vi "Main.vi"(0 "Operations":string(tree), 5 "Path":path=path "C:/Users/khishore.kumar/Khishore/Assignment backups/Assignment 23/SubVI", 7 "Show":bool, 9 "Stop":bool, 11 "Error in":errorcluster) -> (15 "Error out":errorcluster)   [LabVIEW 2020, in "Subpanel access.lvlib"]
doc: "This system will have a file hierarchy to and on double click the panel will be displayed on the subpanel"
uses:
  Subpanel access.lvlib
panel:
  # "SUBPANEL ACCESS"
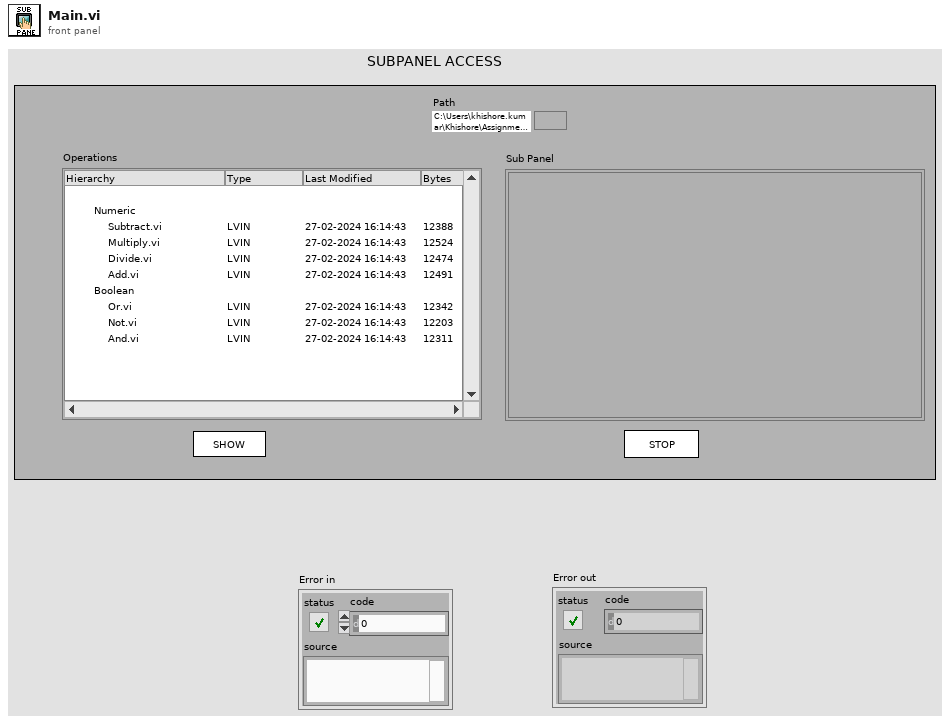
[diagram p1: front panel]
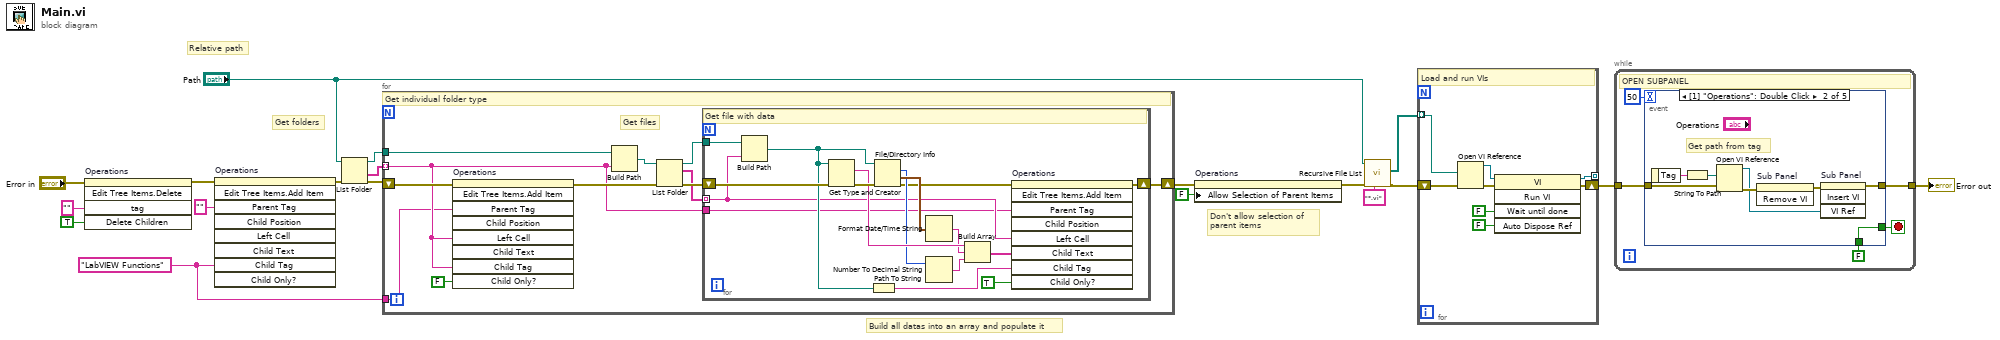
[diagram p0: block diagram]
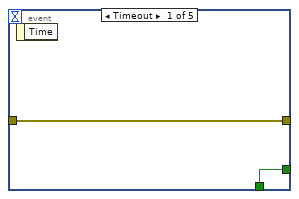
[diagram p2: hidden frame]
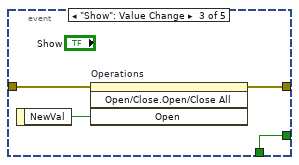
[diagram p3: hidden frame]
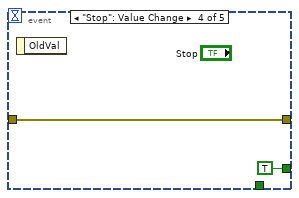
[diagram p4: hidden frame]
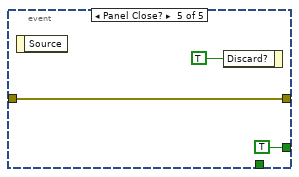
[diagram p5: hidden frame]
diagram:
  w2 = "LabVIEW Functions" ("Child Tag")
  # "Get folders"
  # "Build all datas into an array and populate it"
  # "Relative path"
  # "Don't allow selection of \nparent items"
  n1 = invoke on="Operations" class="Tree (strict)" method="Edit Tree Items.Delete"(error in="Error in", "tag"="" ("Tag"), "Delete Children"=TRUE ("Delete Children?")) -> (error out=w6:errorcluster)  [unwired: 2 in, 4 out]
  n2 = invoke on="Operations" class="Tree (strict)" method="Edit Tree Items.Add Item"(error in=w6, "Parent Tag"="", "Child Tag"=w2) -> (error out=w7:errorcluster)  [unwired: 6 in, 8 out]
  n3 = List Folder(path="Path", error in=w7) -> (path out=w14:path, folder names=w13:string[], error out=w12:errorcluster)  [unwired: 2 in, 1 out]
  n4 = for {
    tunnel: w14 -> [w29]
    shift-right: [w30] -> w5
    shift-left: w12 -> [w23]
    tunnel: w13 -> [w22] mode=indexing
    tunnel: w2 -> [w21]
    # "Get files"
    # "Get individual folder type"
    n5 = invoke on="Operations" class="Tree (strict)" method="Edit Tree Items.Add Item"(error in=w23, "Parent Tag"=w21, "Left Cell"=w22, "Child Tag"=w22, "Child Only?"=FALSE) -> (error out=w24:errorcluster)  [unwired: 4 in, 8 out]
    n6 = Build Path(base path=w29, name or relative path=w22) -> (appended path=w27:path)
    n7 = List Folder(path=w27, error in=w24) -> (path out=w26:path, filenames=w25:string[], error out=w28:errorcluster)  [unwired: 2 in, 1 out]
    n8 = for {
      tunnel: w26 -> [w38]
      tunnel: w22 -> [w31]
      shift-right: [w37] -> w30
      shift-left: w28 -> [w40]
      tunnel: w25 -> [w32] mode=indexing
      # "Get file with data"
      n9 = Build Path(base path=w38, name or relative path=w32) -> (appended path=w39:path)
      n10 = Get Type and Creator(4:w40, 7:w39) -> (0:w46:errorcluster, 2:w45:string)  [unwired: 2 out]
      n11 = Path To String(path=w39) -> (string=w34:string)
      n12 = File/Directory Info(path=w39, error in=w46) -> (size=w42:i64, last mod=w44:timestamp, error out=w36:errorcluster)  [unwired: 4 out]
      n13 = Format Date/Time String(seconds (now)=w44) -> (date/time string=w43:string)  [unwired: 2 in]
      n14 = Number To Decimal String(number=w42) -> (decimal integer string=w41:string)  [unwired: 1 in]
      n15 = Build Array(w45, w43, w41) -> (w33:string[])
      n16 = invoke on="Operations" class="Tree (strict)" method="Edit Tree Items.Add Item"(error in=w36, "Parent Tag"=w31, "Left Cell"=w32, "Child Text"=w33, "Child Tag"=w34, "Child Only?"=TRUE) -> (error out=w37:errorcluster)  [unwired: 3 in, 8 out]
    }
  }
  n17 = property on="Operations" class="Tree (strict)"(error in=w5, "Allow Selection of Parent Items"=FALSE) -> (error out=w4:errorcluster)  [unwired: 1 in, 1 out]
  n18 = call <vilib>:"Recursive File List.vi"("pattern"="*.vi", "error in (no error)"=w4, "Folder Path"="Path") -> ("error out"=w15:errorcluster, "All Files in Dir"=w16:path[])  [unwired: 4 in, 3 out]
  n19 = for {
    tunnel: [w50] -> _ mode=indexing
    shift-right: [w49] -> w17
    shift-left: w15 -> [w47]
    tunnel: w16 -> [w48] mode=indexing
    # "Load and run VIs"
    n20 = Open VI Reference(vi path=w48, error in (no error)=w47) -> (vi reference=w51:refnum<vi>, error out=w52:errorcluster)  [unwired: 4 in]
    n21 = invoke class="VI" method="Run VI"(reference=w51, error in=w52, "Wait until done"=FALSE ("Wait Until Done"), "Auto Dispose Ref"=FALSE ("Auto Dispose Reference")) -> (reference out=w50:refnum<vi>, error out=w49:errorcluster)  [unwired: 1 in, 3 out]
  }
  n22 = while {
    tunnel: w17 -> [w59]
    tunnel: [w57] -> w18
    stop <- w56 stop-if-true
    # "OPEN SUBPANEL"
    n23 = event shown="[1] \"Operations\": Double Click" {
      selector: _ -> [_ _ _ _ _]
      dyn-events: _ -> [_ _ _ _ _]
      timeout: 50 -> [_ _ _ _ _]
      tunnel: w59 -> [w61 w68 w73 w75 w77]
      tunnel: [w61 w69 w72 w75 w77] -> w57
      tunnel: [w60 w62 w70 TRUE TRUE] -> w56
      tunnel: FALSE -> [w60 w62 w70 _ _]
      event Timeout {
        n24 = event-data() -> ()  [unwired: 1 in, 1 out]
      }
      event "Operations": Double Click {
        # "Get path from tag"
        n25 = event-data() -> ("Tag"=w67:string)  [unwired: 1 in]
        n26 = String To Path(string=w67) -> (path=w64:path)
        n27 = Open VI Reference(vi path=w64, error in (no error)=w68) -> (vi reference=w63:refnum<vi>, error out=w65:errorcluster)  [unwired: 4 in]
        n28 = invoke on="Sub Panel" class="SubPnl" method="Remove VI"(error in=w65) -> (error out=w66:errorcluster)  [unwired: 2 in, 2 out]
        n29 = invoke on="Sub Panel" class="SubPnl" method="Insert VI"(error in=w66, "VI Ref"=w63) -> (error out=w69:errorcluster)  [unwired: 2 in, 3 out]
      }
      event "Show": Value Change {
        n30 = event-data() -> ("NewVal"=w71:bool)  [unwired: 1 in]
        n31 = invoke on="Operations" class="Tree (strict)" method="Open/Close.Open/Close All"(error in=w73, "Open"=w71) -> (error out=w72:errorcluster)  [unwired: 2 in, 3 out]
      }
      event "Stop": Value Change {
        n32 = event-data() -> ()  [unwired: 1 in, 1 out]
      }
      event Panel Close? {
        n33 = event-data() -> ()  [unwired: 1 in, 1 out]
        n34 = event-data("Discard?"=TRUE) -> ()  [unwired: 1 in, 1 out]
      }
    }
  }
  "Error out" <- w18
